vi "Launch.vi"(8 "error in (no error)":errorcluster, 9 "Thread ID Pool":refnum<class "Pool ID.lvclass">, 10 "Thread Parameters":refnum<class "Thread Parameters.lvclass">, 11 "Transceiver Thread in":refnum<class "Transceiver Thread.lvclass">) -> (0 "error out":errorcluster, 2 "Interface":refnum<class "Transceiver Interface.lvclass">, 3 "Transceiver Thread out":refnum<class "Transceiver Thread.lvclass">)   [LabVIEW 2017, in "Data Sharing Framework Engine.lvlib" / "Transceiver Thread.lvclass"]
uses:
  Transceiver Thread.lvclass
  Interfaces/Transceiver Interface/Transceiver Interface.lvclass
  old/dsf core/Source/Engine/Classes/Thread Parameters/Thread Parameters.lvclass
  Execution/Pool/Pool ID/Pool ID.lvclass
  Transceiver Thread.lvclass/Transceiver Thread.ctl
  Debug/Debug Flags/Debug Flags.lvclass/Debug Flags.ctl
  Debug/Debug Flags/Debug Flags.lvclass
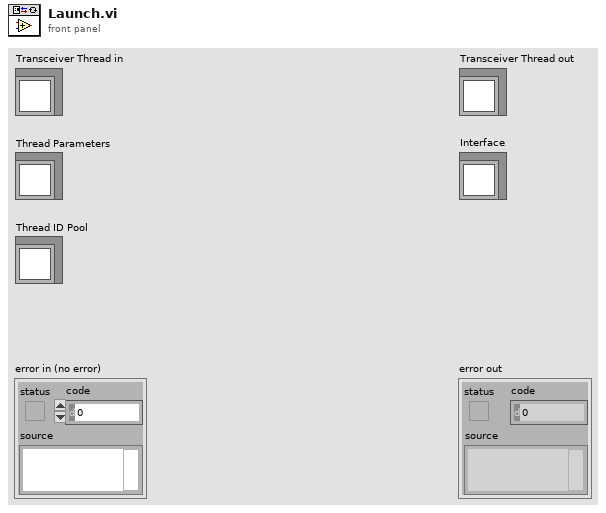
[diagram p1: front panel]
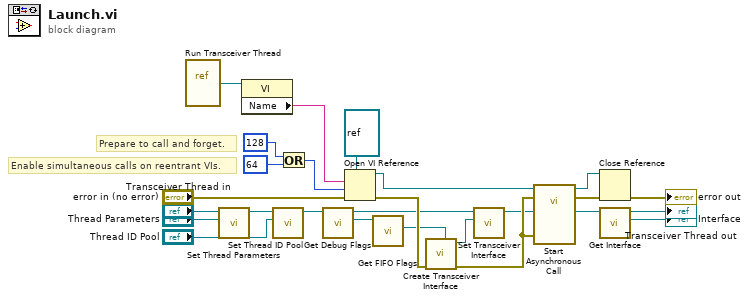
[diagram p0: block diagram]
diagram:
  # "Prepare to call and forget."
  # "Enable simultaneous calls on reentrant VIs."
  n1 = vi-ref "Run Transceiver Thread.vi"() -> (w9:refnum<vi>)
  n2 = call "Set Thread Parameters.vi"("Thread Parameters"="Thread Parameters", "Transceiver Thread in"="Transceiver Thread in") -> ("Transceiver Thread out"=w11:refnum<class "Transceiver Thread.lvclass">)  [unwired: 9 in]
  n3 = property class="VI"(reference=w9) -> ("Name"=w8:string)  [unwired: 1 in, 2 out]
  n4 = call "Set Thread ID Pool.vi"("Thread ID Pool"="Thread ID Pool", "Transceiver Thread in"=w11) -> ("Transceiver Thread out"=w5:refnum<class "Transceiver Thread.lvclass">)  [unwired: 9 in]
  n5 = Or(x=128 ("options"), y=64 ("options")) -> (x .or. y?=w18:i32)
  n6 = call "Get Debug Flags.vi"("Transceiver Thread in"=w5) -> ("Debug Flags"=w4:refnum<class "Debug Flags.lvclass">, "Transceiver Thread out"=w3:refnum<class "Transceiver Thread.lvclass">)  [unwired: 9 in]
  n7 = Open VI Reference(type specifier VI Refnum (for type only)=refnum<vi> refnum, vi path=w8, options=w18, error in (no error)="error in (no error)") -> (vi reference=w23:refnum<vi>, error out=w25:errorcluster)  [unwired: 2 in]
  n8 = call "Get FIFO Flags.vi"("Debug Flags in"=w4) -> ("FIFO"=w6:refnum<class "Debug Flags FIFO.lvclass">)  [unwired: 9 in, 1 out]
  n9 = call "Create Transceiver Interface.vi"("FIFO Debug Flags"=w6, "error in (no error)"=w25) -> ("error out"=w2:errorcluster, "Transceiver Interface"=w7:refnum<class "Transceiver Interface.lvclass">)  [unwired: 8 in]
  n10 = call "Set Transceiver Interface.vi"("Interface"=w7, "Transceiver Thread in"=w3) -> ("Transceiver Thread out"=w1:refnum<class "Transceiver Thread.lvclass">)  [unwired: 9 in]
  n11 = call-by-ref "Start Asynchronous Call"(reference=w23, error in=w2, 8:"error in (no error)"=w2, "Transceiver Thread in"=w1) -> (reference out=w21:refnum<vi>, error out=w22:errorcluster)  [unwired: 8 in, 2 out]
  n12 = Close Reference(reference=w21, error in (no error)=w22) -> (error out=→"error out":errorcluster)
  n13 = call "Get Interface.vi"("Transceiver Thread in"=w1) -> ("Interface"=→"Interface":refnum<class "Transceiver Interface.lvclass">, "Transceiver Thread out"=→"Transceiver Thread out":refnum<class "Transceiver Thread.lvclass">)  [unwired: 9 in]
